vi "Keithley 27XX Temperature (Thermocouple).vi"() -> ()   [LabVIEW 2020]
doc: "This example VI shows how to use thermocouples to take a temperature measurement.\n\nNote:\nFor front panel measurements, make sure the Input switch is in the out position(F)\nFor plug-in card measurements, make sure the Input switch is in the in poisition(R)"
uses:
  <instrlib>/Keithley 27XX/Public/Configure/Measurement Specific/Configure Thermocouple.vi
  <instrlib>/Keithley 27XX/Public/Data/Read Single Point.vi
  <instrlib>/Keithley 27XX/Public/Data/Read Multiple Direct.vi
  <instrlib>/Keithley 27XX/Keithley 27XX.lvlib
panel:
  in  "Delay ms":ext=23.0
  in  "deney no":string
  out "appended path":path
  in  "Temperature (0: Celsius)":u16(ring) items=["Celsius", "Fahrenheit", "Kelvin"]
  in  "VISA resource name":refnum<visa-resource-name>
  in  "Tab Control":enum32{"single channel", "multi channel"}(tab)
  out "Waveform Chart":dbl(graph)
  in  "Thermocouple Type (1: K)":u16(ring)=1 items=["J", "K", "T", "E", "R", "S", "B", "N"]
  in  "Reference Junction Type (0: Simulated)":u16(ring) items=["Simulated", "Internal", "External"]
  in  "Simulated Refence Temperature (23)":dbl=23.0
  in  "Channel (101)":string="101"
  out "Measurement Data":dbl
  in  "Sample Count (100)":i32=100
  in  "Start":bool
  in  "stop 2":bool
  in  "Save Button 2":bool
  in  "Save Button":bool
  out "Table":string[][](table)
  out "Channel":string[](array[string])
  out "Measurement Data":dbl[](array[numeric])
  in  "Thermocouple Type (1: K) 2":u16(ring)=1 items=["J", "K", "T", "E", "R", "S", "B", "N"]
  in  "Sample Count (100) 2":i32=100
  in  "Reference Junction Type\n (0: Simulated)  2":u16(ring) items=["Simulated", "Internal", "External"]
  in  "Simulated Reference \nTemperature (23 deg C)":dbl=23.0
  in  "Enable Open Detector? (False)":bool
  in  "Channel":string[](array[string])
  in  "All Data Elements (False)":bool
  in  "stop 3":bool
  in  "Start 2":bool
  in  "Serial Configuration":T1={"Baud Rate (9600)"=9600, "Flow Control (1: XON/XOFF)"=1, "Termination Char (0:CR)"=0} {"Termination Char (0:CR)" items=["CR", "LF", "CRLF (Do not use)", "LFCR (Do not use)"]; "Flow Control (1: XON/XOFF)" items=["None", "XON/XOFF", "RTS/CTS (2701 Only)", "XON/XOFF & RTS/CTS (2701 Only)"]; "Baud Rate (9600)" items=["300"=300, "600"=600, "1200"=1200, "2400"=2400, "4800"=4800, "9600"=9600, "19.2k"=19200, "38.4k (2701 Only)"=38400, "57.6k (2701 Only)"=57600, "115.2k (2701 Only)"=115200]}
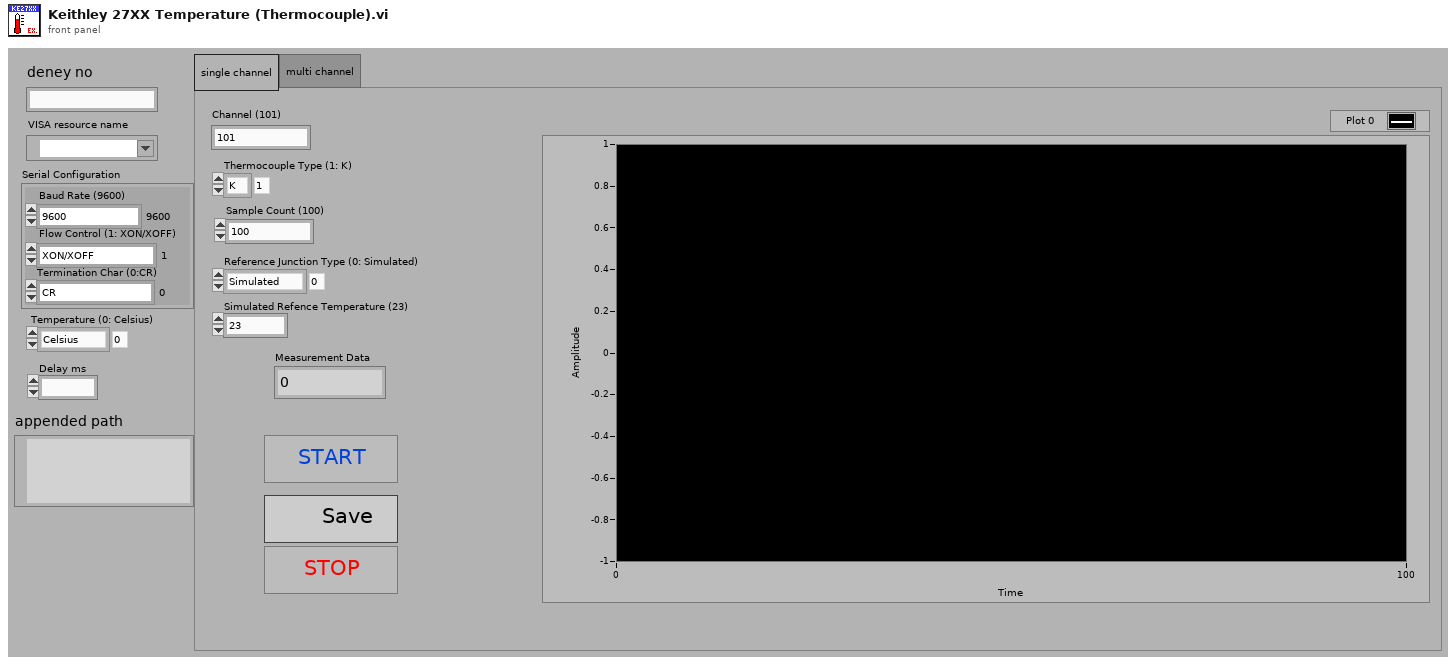
[diagram p1: front panel]
types:
  T1 = cluster{"Baud Rate (9600)":u32, "Flow Control (1: XON/XOFF)":u16, "Termination Char (0:CR)":u16}
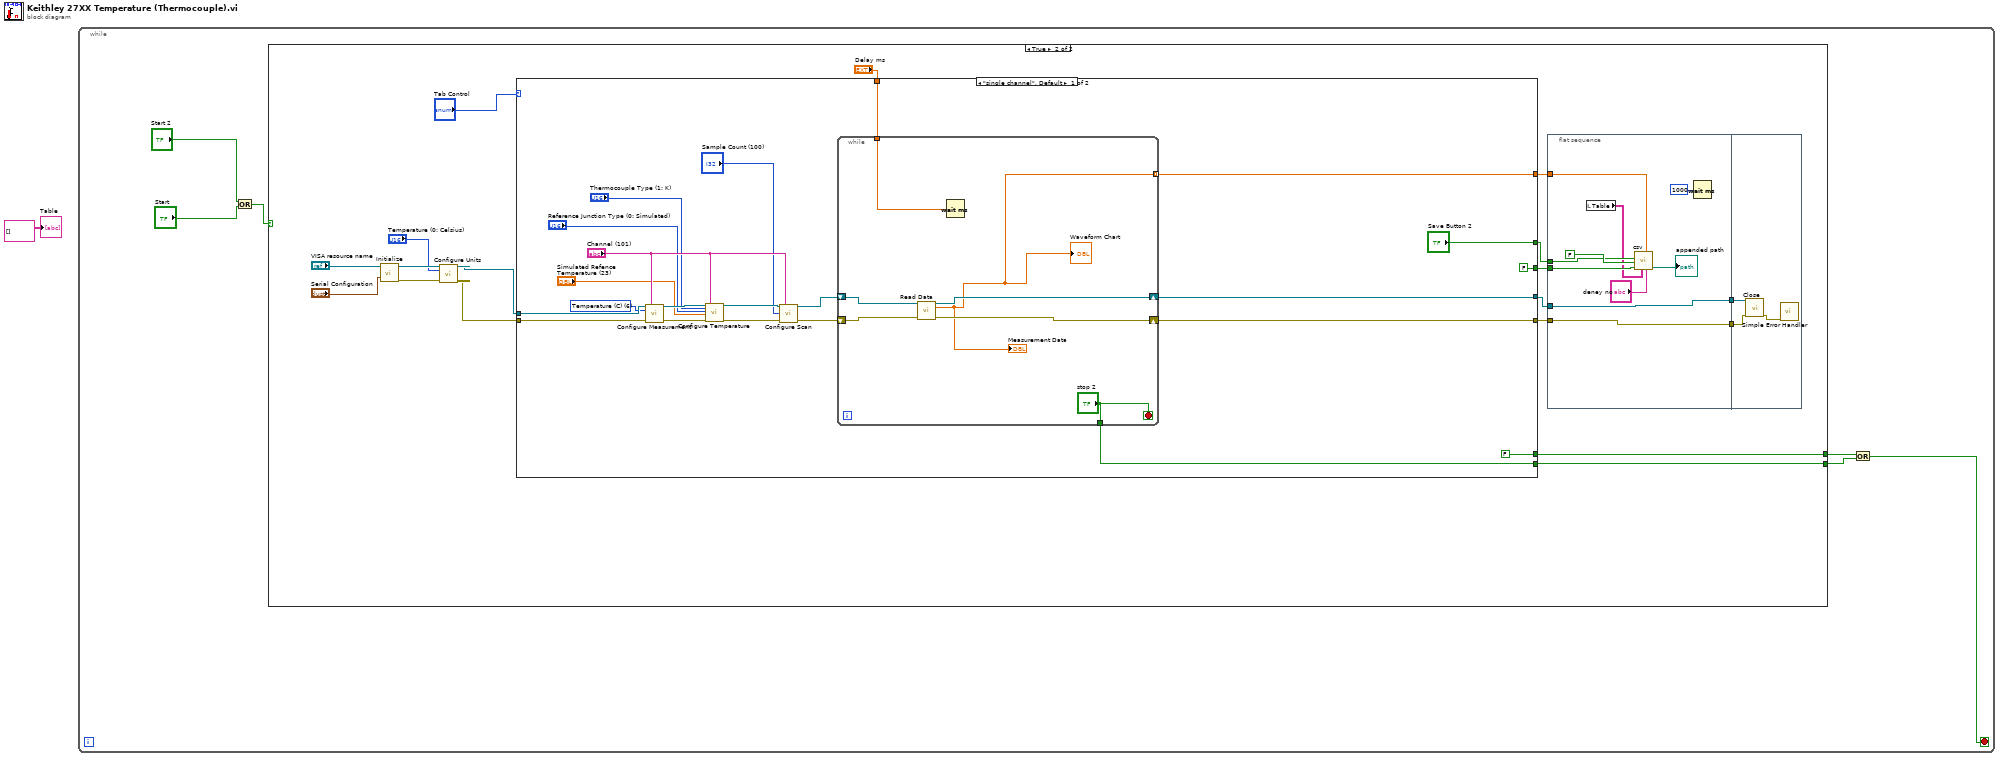
[diagram p0: block diagram]
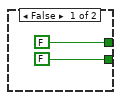
[diagram p2: hidden frame]
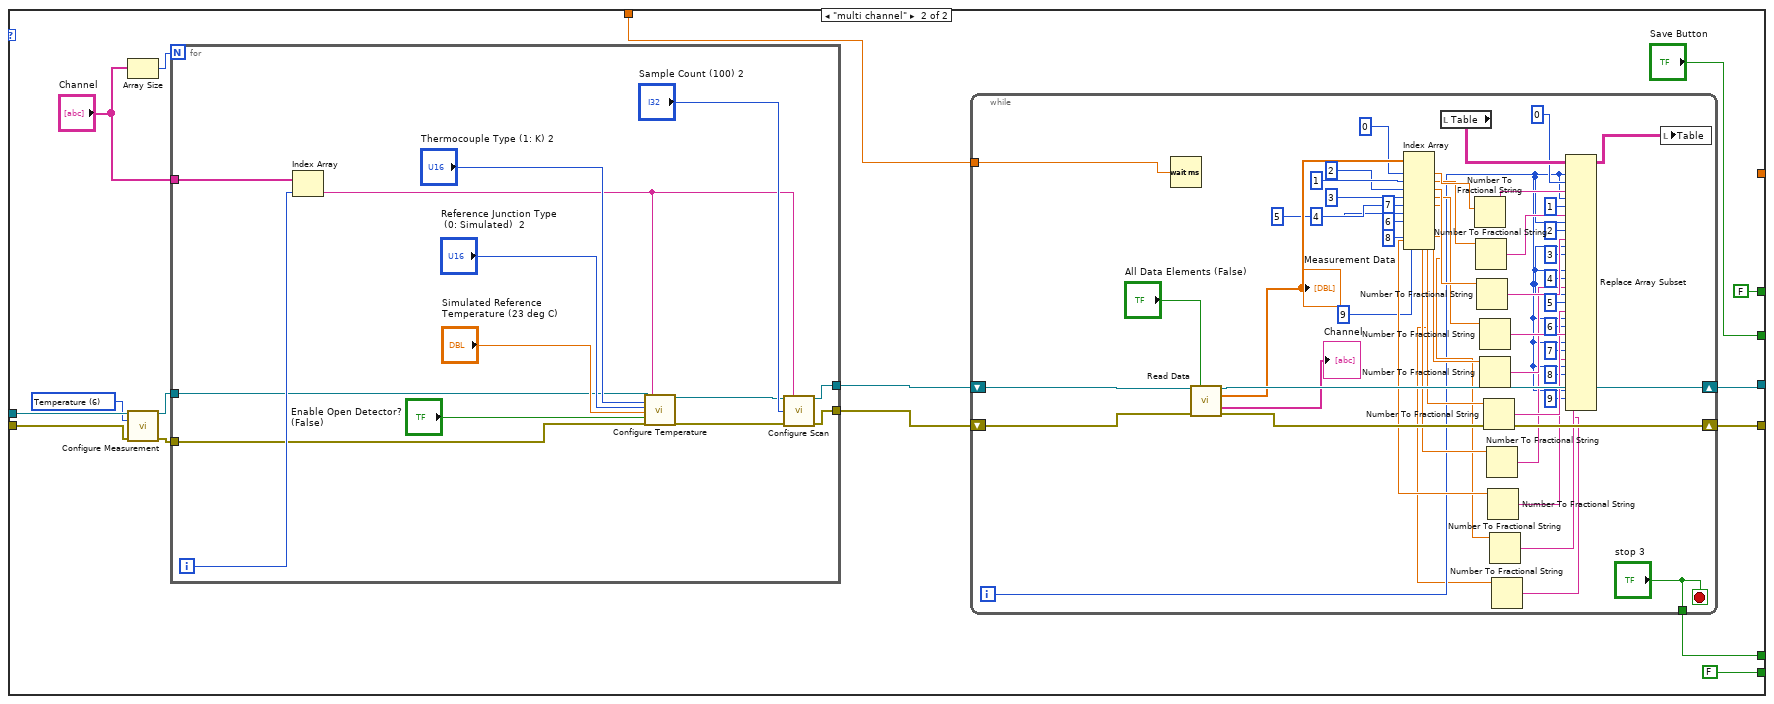
[diagram p3: hidden frame]
diagram:
  n1 = while {
    stop <- w5 stop-if-true
    n2 = Or(x="Start 2", y="Start") -> (x .or. y?=w2:bool)
    n3 = case shown="True" w2 {
      tunnel: [FALSE ("stop 3") w18] -> w7
      tunnel: [FALSE ("stop 2") w17] -> w6
      frame False {
      }
      frame True {
        n4 = call <instrlib>:"Initialize.vi"("VISA resource name"="VISA resource name", "Serial Configuration"="Serial Configuration") -> ("VISA resource name out"=w27:refnum<visa-resource-name>, "error out"=w24:errorcluster)  [unwired: 12 in]
        n5 = call <instrlib>:"Configure Units.vi"("VISA resource name"=w27, "Temperature (0: Celsius)"="Temperature (0: Celsius)", "error in (no error)"=w24) -> ("VISA resource name out"=w21:refnum<visa-resource-name>, "error out"=w20:errorcluster)  [unwired: 11 in]
        n6 = case shown="\"single channel\", Default" "Tab Control" {
          tunnel: w21 -> [w52 w85]
          tunnel: w20 -> [w50 w84]
          tunnel: [w49 w81] -> w13
          tunnel: [w48 w82] -> w10
          tunnel: "Delay ms" -> [w46 w74]
          tunnel: [FALSE ("stop 3") w73] -> w18
          tunnel: [w44 FALSE ("stop 2")] -> w17
          tunnel: [FALSE ("Save Button") "Save Button"] -> w16
          tunnel: ["Save Button 2" FALSE ("Save Button 2")] -> w15
          tunnel: [w41 _] -> w14
          frame "single channel", Default {
            w51 = u16 6 items=["DC Voltage", "AC Voltage", "DC Current", "AC Current", "Resistance", "Four-Wire Resistance", "Temperature (C)", "Frequency", "Period", "Continuity"] ("Function (0: DC Voltage)")
            n7 = call <instrlib>:"Configure Measurement.vi"("VISA resource name"=w52, "Scan List (Empty)"="Channel (101)", "Function (0: DC Voltage)"=w51, "error in (no error)"=w50) -> ("VISA resource name out"=w62:refnum<visa-resource-name>, "error out"=w53:errorcluster)  [unwired: 10 in]
            n8 = call-poly <instrlib>:"Configure Temperature.vi"("VISA resource name"=w62, "Thermocouple Type (1: K)"="Thermocouple Type (1: K)", "Reference Junction Type (0: Simulated)"="Reference Junction Type (0: Simulated)", "Simulated Reference Temperature (23 deg C)"="Simulated Refence Temperature (23)", "error in (no error)"=w53, "Scan List (Empty)"="Channel (101)") -> ("VISA resource name out"=w57:refnum<visa-resource-name>, "error out"=w58:errorcluster)  [unwired: 12 in]
            n9 = call <instrlib>:"Configure Scan.vi"("VISA resource name"=w57, "Channel List (101:110)"="Channel (101)", "Sample Count (100)"="Sample Count (100)", "error in (no error)"=w58) -> ("VISA resource name out"=w60:refnum<visa-resource-name>, "error out"=w59:errorcluster)  [unwired: 10 in]
            n10 = while {
              shift-right: [w67] -> w49
              shift-left: w60 -> [w69]
              shift-right: [w66] -> w48
              shift-left: w59 -> [w68]
              tunnel: w46 -> [w65]
              tunnel: ["stop 2"] -> w44
              tunnel: [w63] -> w41 mode=indexing
              stop <- "stop 2" stop-if-true
              n11 = call-poly <instrlib>:"Read Data.vi"("VISA resource name"=w69, "error in (no error)"=w68) -> ("VISA resource name out"=w67:refnum<visa-resource-name>, "Measurement Data"=w63:dbl, "error out"=w66:errorcluster)  [unwired: 11 in]
              "Measurement Data" <- w63
              "Waveform Chart" <- w63
              n12 = Wait (ms)(milliseconds to wait=w65) -> ()  [unwired: 1 out]
            }
          }
          frame "multi channel" {
            w83 = u16 6 items=["DC Voltage", "AC Voltage", "DC Current", "AC Current", "Resistance", "Four-Wire Resistance", "Temperature", "Frequency", "Period", "Continuity"] ("Function (0: DC Voltage)")
            n13 = Array Size(array="Channel") -> (size(s)=w80:i32)
            n14 = call <instrlib>:"Configure Measurement.vi"("VISA resource name"=w85, "Function (0: DC Voltage)"=w83, "error in (no error)"=w84) -> ("VISA resource name out"=w78:refnum<visa-resource-name>, "error out"=w77:errorcluster)  [unwired: 11 in]
            n15 = for {
              N: w80 -> [_]
              tunnel: "Channel" -> [w144]
              tunnel: w78 -> [w141]
              tunnel: w77 -> [w140]
              tunnel: [w139] -> w76
              tunnel: [w138] -> w75
              i -> [w143]
              n16 = Index Array(array=w144, index=w143) -> (element=w142:string)
              n17 = call-poly <instrlib>:"Configure Temperature.vi"("VISA resource name"=w141, "Thermocouple Type (1: K)"="Thermocouple Type (1: K) 2", "Reference Junction Type (0: Simulated)"="Reference Junction Type\n (0: Simulated)  2", "Simulated Reference Temperature (23 deg C)"="Simulated Reference \nTemperature (23 deg C)", "Enable Open Detector? (False)"="Enable Open Detector? (False)", "error in (no error)"=w140, "Scan List (Empty)"=w142) -> ("VISA resource name out"=w146:refnum<visa-resource-name>, "error out"=w145:errorcluster)  [unwired: 11 in]
              n18 = call <instrlib>:"Configure Scan.vi"("VISA resource name"=w146, "Channel List (101:110)"=w142, "Sample Count (100)"="Sample Count (100) 2", "error in (no error)"=w145) -> ("VISA resource name out"=w139:refnum<visa-resource-name>, "error out"=w138:errorcluster)  [unwired: 10 in]
            }
            n19 = while {
              shift-right: [w136] -> w81
              shift-left: w76 -> [w135]
              shift-right: [w137] -> w82
              shift-left: w75 -> [w134]
              tunnel: w74 -> [w131]
              tunnel: ["stop 3"] -> w73
              i -> [w90]
              stop <- "stop 3" stop-if-true
              n20 = Wait (ms)(milliseconds to wait=w131) -> ()  [unwired: 1 out]
              n21 = call-poly <instrlib>:"Read Data.vi"("VISA resource name"=w135, "All Data Elements (False)"="All Data Elements (False)", "error in (no error)"=w134) -> ("VISA resource name out"=w136:refnum<visa-resource-name>, "Measurement Data"=w130:dbl[], "Channel"=→"Channel":string[], "error out"=w137:errorcluster)  [unwired: 7 in, 2 out]
              "Measurement Data" <- w130
              n22 = Index Array(array=w130, index #1=0 ("index"), index #2=1 ("index"), index #3=2 ("index"), index #4=3 ("index"), index #5=4 ("index"), index #6=5 ("index"), index #7=6 ("index"), index #8=7 ("index"), index #9=8 ("index"), index #10=9 ("index")) -> (element #1=w125:dbl, element #2=w122:dbl, element #3=w117:dbl, element #4=w113:dbl, element #5=w109:dbl, element #6=w105:dbl, element #7=w101:dbl, element #8=w97:dbl, element #9=w93:dbl, element #10=w87:dbl)
              n23 = local read "Table"() -> (w129:string[][])
              n24 = Number To Fractional String(number=w125) -> (F-format string=w124:string)  [unwired: 3 in]
              n25 = Number To Fractional String(number=w122) -> (F-format string=w121:string)  [unwired: 3 in]
              n26 = Number To Fractional String(number=w117) -> (F-format string=w116:string)  [unwired: 3 in]
              n27 = Number To Fractional String(number=w113) -> (F-format string=w112:string)  [unwired: 3 in]
              n28 = Number To Fractional String(number=w109) -> (F-format string=w108:string)  [unwired: 3 in]
              n29 = Number To Fractional String(number=w105) -> (F-format string=w104:string)  [unwired: 3 in]
              n30 = Number To Fractional String(number=w101) -> (F-format string=w100:string)  [unwired: 3 in]
              n31 = Number To Fractional String(number=w97) -> (F-format string=w96:string)  [unwired: 3 in]
              n32 = Number To Fractional String(number=w93) -> (F-format string=w92:string)  [unwired: 3 in]
              n33 = Number To Fractional String(number=w87) -> (F-format string=w88:string)  [unwired: 3 in]
              n34 = Replace Array Subset(array=w129, new element #1=w124, index (row) #1=w90, index (col) #1=0 ("disabled index (col)"), new element #2=w121, index (row) #2=w90, index (col) #2=1 ("disabled index (col)"), new element #3=w116, index (row) #3=w90, index (col) #3=2 ("disabled index (col)"), new element #4=w112, index (row) #4=w90, index (col) #4=3 ("disabled index (col)"), new element #5=w108, index (row) #5=w90, index (col) #5=4 ("disabled index (col)"), new element #6=w104, index (row) #6=w90, index (col) #6=5 ("disabled index (col)"), new element #7=w100, index (row) #7=w90, index (col) #7=6 ("disabled index (col)"), new element #8=w96, index (row) #8=w90, index (col) #8=7 ("disabled index (col)"), new element #9=w92, index (row) #9=w90, index (col) #9=8 ("disabled index (col)"), new element #10=w88, index (row) #10=w90, index (col) #10=9 ("disabled index (col)")) -> (w128:string[][])
              n35 = local write "Table"(w128) -> ()
            }
          }
        }
        n36 = flat-sequence {
          tunnel: w16 -> [w37]
          tunnel: w15 -> [w35]
          tunnel: w14 -> [w29]
          tunnel: w13 -> [w32]
          tunnel: [w32] -> w12
          tunnel: [w31] -> w11
          tunnel: w10 -> [w31]
          tunnel: w12 -> [w39]
          tunnel: w11 -> [w38]
          frame #0 {
            n37 = local read "Table"() -> (w28:string[][])
            n38 = call "csv.vi"("deney no"="deney no", "1D data"=w29, "Table Control"=w28, "Boolean-String"=w37, "Boolean-Namber"=FALSE, "Boolean-Namber 1D"=w35) -> ("appended path"=→"appended path":path)  [unwired: 2 in, 3 out]
            n39 = Wait (ms)(milliseconds to wait=u32 1000) -> ()  [unwired: 1 out]
          }
          frame #1 {
            n40 = call <instrlib>:"Close.vi"("VISA resource name"=w39, "error in (no error)"=w38) -> ("error out"=w40:errorcluster)  [unwired: 13 in]
            n41 = call <vilib>:"Simple Error Handler.vi"("error in (no error)"=w40) -> ()  [unwired: 4 in, 5 out]
          }
        }
      }
    }
    n42 = Or(x=w7, y=w6) -> (x .or. y?=w5:bool)
  }
  "Table" <- string[][] [] ("Table")
